vi "Populate File Tree.vi"(7 "Tree Refnum":refnum<vi>, 8 "error in (no error)":errorcluster, 9 "Diff'd Parent String/Tag":string="/", 10 "Tree":string(tree), 11 "Folder Array In":string[](array[string])) -> (0 "error out":errorcluster, 2 "Folder Names Array Out":string[](array[string]))   [LabVIEW 2023]
panel:
  out "Test Values":string[](array[string])
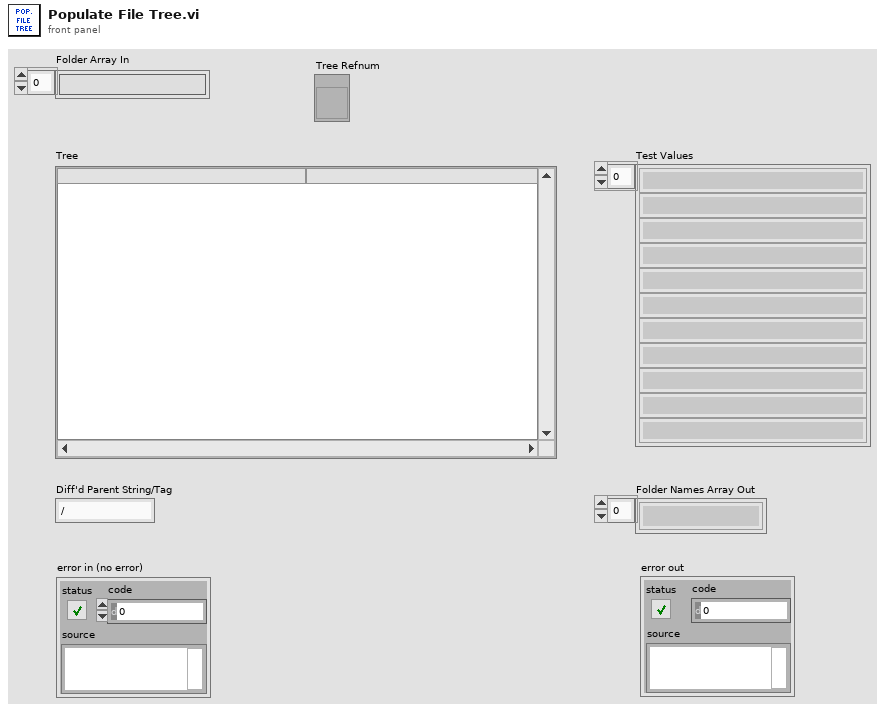
[diagram p1: front panel]
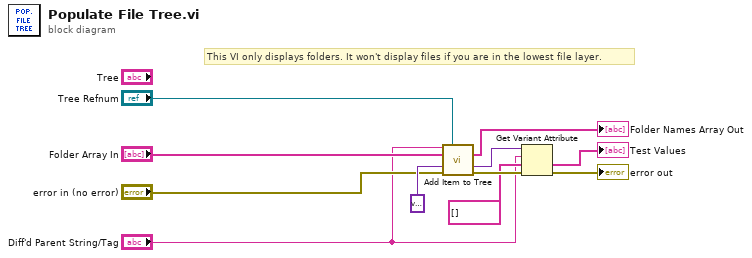
[diagram p0: block diagram]
diagram:
  # "This VI only displays folders. It won't display files if you are in the lowest file layer."
  n1 = call "Add Item to Tree.vi"("Parent Tag Name In"="Diff'd Parent String/Tag", "TreeControl in"="Tree Refnum", "File/Folder Names Array"="Folder Array In", "variant in"=variant, "error in (no error)"="error in (no error)") -> ("Dup File/Folder Names Array"=→"Folder Names Array Out":string[], "variant out"=w9:variant, "error out"=w8:errorcluster)  [unwired: 7 in, 1 out]
  n2 = Get Variant Attribute(Variant=w9, name="Diff'd Parent String/Tag", default value (empty Variant)=string[] [], error in=w8) -> (value=→"Test Values":string[], error out=→"error out":errorcluster)  [unwired: 2 out]
